vi "Update DTC Active Values.vi"(8 "error in":errorcluster, 11 "Simulated Addresses in":T1[](array[typedef]) {"Simulated Addresses"."J1939 XNET Settings"."Name" format="%.0x"; "Simulated Addresses"."DM1 Data"."Data Reference" format="%.0x"; "Simulated Addresses"."DM1 Active?"."Data Reference" format="%.0x"; "Simulated Addresses"."DM2 Data"."Data Reference" format="%.0x"; "Simulated Addresses"."DM2 Active?"."Data Reference" format="%.0x"}) -> (0 "error out":errorcluster, 3 "Simulated Addresses out":T1[](array[typedef]) {"Simulated Addresses"."J1939 XNET Settings"."Name" format="%.0x"; "Simulated Addresses"."DM1 Data"."Data Reference" format="%.0x"; "Simulated Addresses"."DM1 Active?"."Data Reference" format="%.0x"; "Simulated Addresses"."DM2 Data"."Data Reference" format="%.0x"; "Simulated Addresses"."DM2 Active?"."Data Reference" format="%.0x"})   [LabVIEW 2013, in "J1939 Addon Engine.lvlib"]
uses:
  Types/Simulated Settings.ctl
  Shared/Types/Compiled Simulated Settings.ctl
  Shared/Types/Monitor Settings.ctl
  <vilib>/NI Veristand/Custom Device API/Block Data Reference.ctl
  <vilib>/NI Veristand/Custom Device API/Data Reference.ctl
  Types/DTC FIFOs.ctl
  <vilib>/NI Veristand/Custom Device API/Global Data Refs.vi
  J1939 Addon Engine.lvlib
  <vilib>/NI Veristand/Custom Device API/Custom Device API.lvlib
  Shared/J1939 Addon Shared.lvlib
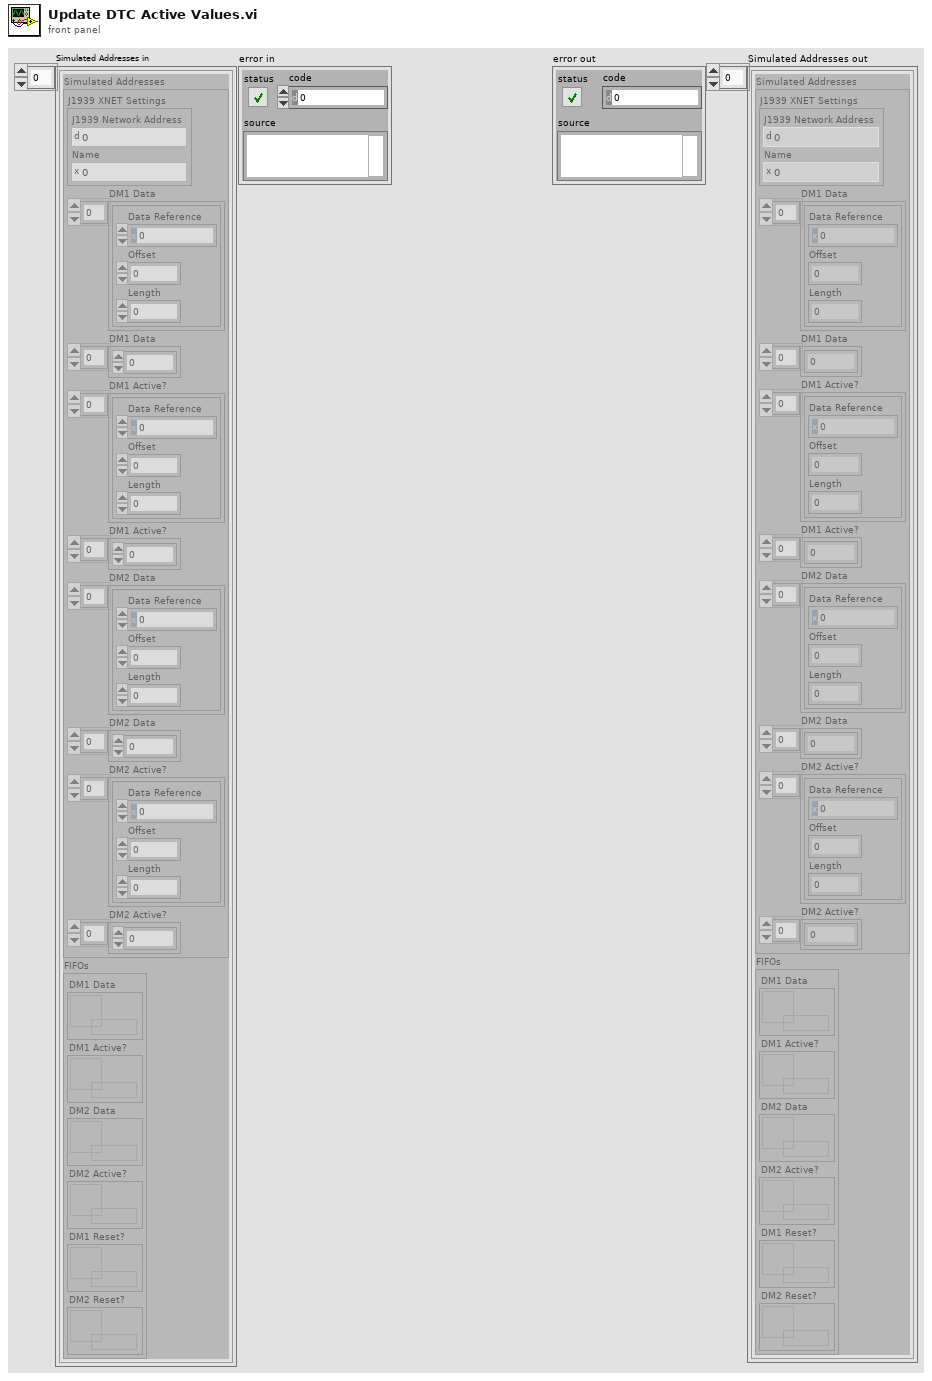
[diagram p1: front panel]
types:
  T1 = typedef "J1939 Addon Engine.lvlib/Simulated Settings.ctl" = cluster{"Simulated Addresses":T2, "FIFOs":T6}
  T2 = typedef "J1939 Addon Shared.lvlib/Compiled Simulated Settings.ctl" = cluster{"J1939 XNET Settings":T3, "DM1 Data":T4[], "DM1 Data":dbl[], "DM1 Active?":T4[], "DM1 Active?":dbl[], "DM2 Data":T4[], "DM2 Data":dbl[], "DM2 Active?":T4[], "DM2 Active?":dbl[]}
  T3 = typedef "J1939 Addon Shared.lvlib/Monitor Settings.ctl" = cluster{"J1939 Network Address":u8, "Name":u64}
  T4 = typedef "Custom Device API.lvlib/Block Data Reference.ctl" = cluster{"Data Reference":T5, "Offset":i32, "Length":i32}
  T5 = typedef "Custom Device API.lvlib/Data Reference.ctl" = i32
  T6 = typedef "J1939 Addon Engine.lvlib/DTC FIFOs.ctl" = cluster{"DM1 Data":refnum<k33>, "DM1 Active?":refnum<k33>, "DM2 Data":refnum<k33>, "DM2 Active?":refnum<k33>, "DM1 Reset?":refnum<k33>, "DM2 Reset?":refnum<k33>}
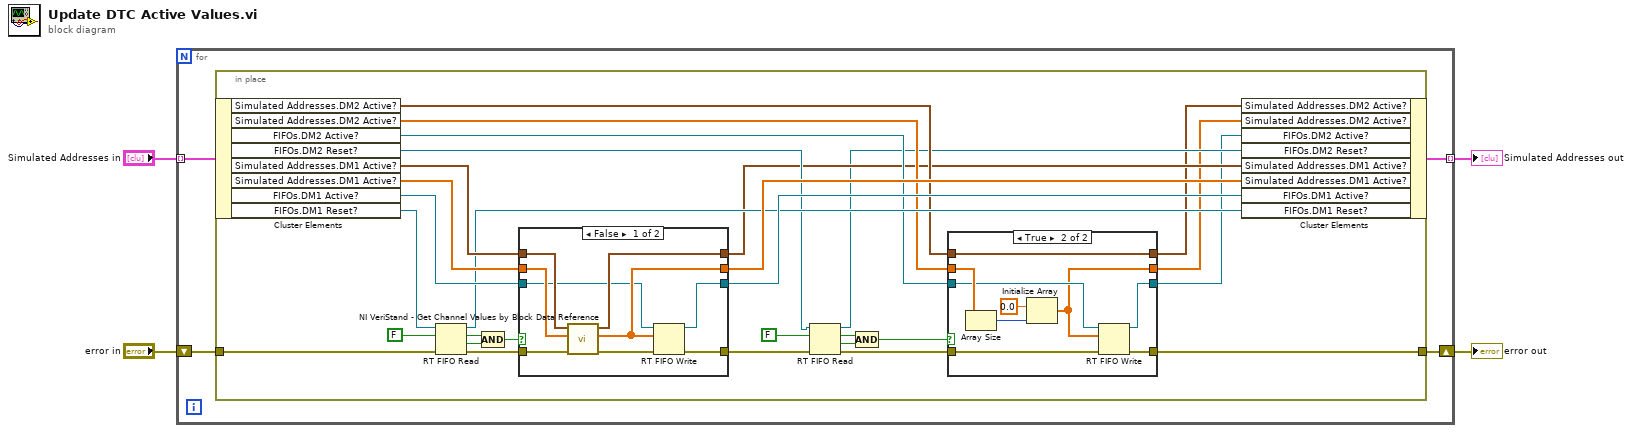
[diagram p0: block diagram]
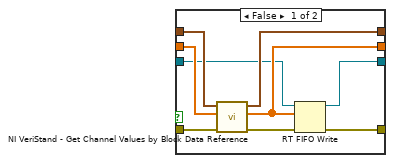
[diagram p2: hidden frame]
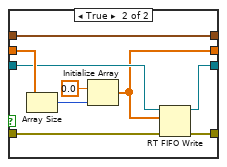
[diagram p3: hidden frame]
diagram:
  n1 = for {
    tunnel: "Simulated Addresses in" -> [w8] mode=indexing
    shift-right: [w7] -> w2
    shift-left: "error in" -> [w5]
    tunnel: [w6] -> w1 mode=indexing
    n2 = in-place {
      in-place-border: [w10] -> w7
      in-place-border: w5 -> [w9]
      n3 = in-place-cluster #1(w8) -> ("Simulated Addresses.DM2 Active?"=w16:T4[], "Simulated Addresses.DM2 Active?"=w17:dbl[], "FIFOs.DM2 Active?"=w18:refnum<k33>, "FIFOs.DM2 Reset?"=w19:refnum<k33>, "Simulated Addresses.DM1 Active?"=w32:T4[], "Simulated Addresses.DM1 Active?"=w31:dbl[], "FIFOs.DM1 Active?"=w29:refnum<k33>, "FIFOs.DM1 Reset?"=w37:refnum<k33>)
      n4 = RT FIFO Read(0:w37, 1:FALSE ("element"), 3:w9) -> (8:w20:refnum<k33>, 9:w36:bool, 10:w35:bool, 11:w30:errorcluster)  [unwired: 1 in, 1 out]
      n5 = Compound Arithmetic op=AND(w36, w35) -> (w33:bool)
      n6 = case shown="False" w33 {
        tunnel: w32 -> [w64 w65]
        tunnel: w31 -> [w63 w72]
        tunnel: w30 -> [w62 w73]
        tunnel: w29 -> [w57 w69]
        tunnel: [w60 w66] -> w28
        tunnel: [w59 w68] -> w23
        tunnel: [w56 w67] -> w27
        tunnel: [w58 w65] -> w15
        frame False {
          n7 = call <vilib>:"NI VeriStand - Get Channel Values by Block Data Reference.vi"("error in (no error)"=w62, "Values Array in"=w63, "Block Data Ref"=w64) -> ("error out"=w61:errorcluster, "Values Array out"=w60:dbl[], "Block Data Ref dup"=w58:T4[])  [unwired: 6 in]
          n8 = RT FIFO Write(0:w57, 1:w60, 3:w61) -> (8:w56:refnum<k33>, 11:w59:errorcluster)  [unwired: 2 in, 2 out]
        }
        frame True {
          n9 = Array Size(array=w72) -> (size(s)=w71:i32)
          n10 = Initialize Array(0.0 ("element"), w71) -> (w66:dbl[])
          n11 = RT FIFO Write(0:w69, 1:w66, 3:w73) -> (8:w67:refnum<k33>, 11:w68:errorcluster)  [unwired: 2 in, 2 out]
        }
      }
      n12 = RT FIFO Read(0:w19, 1:FALSE ("element"), 3:w23) -> (8:w14:refnum<k33>, 9:w24:bool, 10:w25:bool, 11:w22:errorcluster)  [unwired: 1 in, 1 out]
      n13 = Compound Arithmetic op=AND(w24, w25) -> (w21:bool)
      n14 = case shown="True" w21 {
        tunnel: w16 -> [w46 w47]
        tunnel: w17 -> [w45 w54]
        tunnel: w22 -> [w44 w55]
        tunnel: w18 -> [w39 w51]
        tunnel: [w42 w48] -> w12
        tunnel: [w41 w50] -> w10
        tunnel: [w38 w49] -> w11
        tunnel: [w40 w47] -> w13
        frame False {
          n15 = call <vilib>:"NI VeriStand - Get Channel Values by Block Data Reference.vi"("error in (no error)"=w44, "Values Array in"=w45, "Block Data Ref"=w46) -> ("error out"=w43:errorcluster, "Values Array out"=w42:dbl[], "Block Data Ref dup"=w40:T4[])  [unwired: 6 in]
          n16 = RT FIFO Write(0:w39, 1:w42, 3:w43) -> (8:w38:refnum<k33>, 11:w41:errorcluster)  [unwired: 2 in, 2 out]
        }
        frame True {
          n17 = Array Size(array=w54) -> (size(s)=w53:i32)
          n18 = Initialize Array(0.0 ("element"), w53) -> (w48:dbl[])
          n19 = RT FIFO Write(0:w51, 1:w48, 3:w55) -> (8:w49:refnum<k33>, 11:w50:errorcluster)  [unwired: 2 in, 2 out]
        }
      }
      n20 = in-place-cluster #1("Simulated Addresses.DM2 Active?"=w13, "Simulated Addresses.DM2 Active?"=w12, "FIFOs.DM2 Active?"=w11, "FIFOs.DM2 Reset?"=w14, "Simulated Addresses.DM1 Active?"=w15, "Simulated Addresses.DM1 Active?"=w28, "FIFOs.DM1 Active?"=w27, "FIFOs.DM1 Reset?"=w20) -> (w6:T1)
    }
  }
  "error out" <- w2
  "Simulated Addresses out" <- w1
